vi "SiemensDigitalEnergyMeter.vi"() -> ()   [LabVIEW 2018, in "Visualization.lvlib" / "VisualizeSensor.lvclass"]
doc: "This VI listens for any measurement data associated with the provided PluginName and displays it to the user for analysis. The display is only suitable for data coming from the Siemens Plugin."
uses:
  VisualizeSensor.lvclass
  VisualizeBase/VisualizeBase_class/SubVIs/VisualizationOptions.ctl
  <vilib>/Utility/miscctls.llb/LVRectTypeDef.ctl
  Sensor/SensorShared/clSensorData.ctl
  <extravilib>/ChannelInstances/Tag-bool/Write With Abort.vi
  <extravilib>/ChannelInstances/Tag-bool/Read With Abort.vi
  <extravilib>/ChannelInstances/Tag-bool/Instantiate.vi
  <extravilib>/ChannelInstances/Tag-bool/EndpointRead.vi
  <vilib>/Utility/error.llb/Error Cluster From Error Code.vi
  <extravilib>/ChannelInstances/Tag-bool/Endpoint.vi
  <vilib>/ErrorRing/Error Ring.xnode
  <userlib>/NIST/NISTErrorLib/NISTErrorLib.lvlib
  VisualizeBase/VisualizeBase_class/VisualizeBase.lvclass
  Sensor/SensorShared/SensorShared.lvlib
  Sensor/SensorModule/SensorModule.lvlib
  <extravilib>/ChannelInstances/Tag-bool.lvlib
  TestClass/Test.lvclass
  StatusAndLog/VisualizeStatus.lvclass
panel:
  in  "btnPause":bool=TRUE
  out "VisualizationProperties":T1={"PauseAtStartup"=TRUE, "LogData"=FALSE, "LaunchInSubPanel"=TRUE, "FPMonitor"=0, "FPWindowBounds"={"Left"=0, "Top"=0, "Right"=0, "Bottom"=0}, "MonitorBounds"={"Left"=0, "Top"=0, "Right"=0, "Bottom"=0}}
  in  "INIFilePath":path
  in  "ModuleID":i32
  in  "Log Data":bool=TRUE
  in  "btnStop":bool
  in  "btnReset":bool
  in  "btnClearTest":bool
  out "Siemens":waveform(dbl)[](graph)=[{"t0"=timestamp(3657200531.6397257 s since 1904-01-01), "dt"=1.0, "Y"=[46.19]}, {"t0"=timestamp(3657200531.6397257 s since 1904-01-01), "dt"=1.0, "Y"=[2.0]}, {"t0"=timestamp(3657200531.6397257 s since 1904-01-01), "dt"=1.0, "Y"=[60.0]}]
  out "ErrorArray":errorcluster[](array[cluster])
  out "Incorrect DataType?":bool
  out "String Results":string="Sensor.RoomAlert1"
  in  "PluginName":string="Sensor.RoomAlert1"
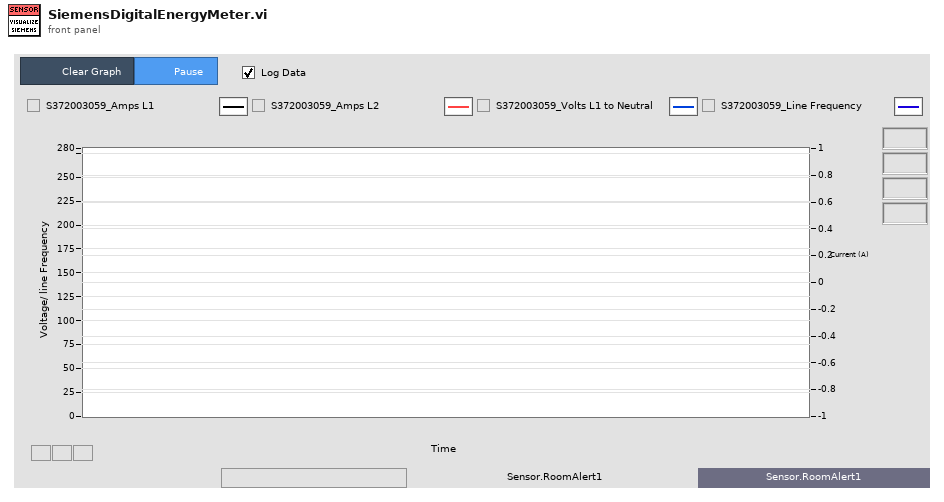
[diagram p1: front panel]
types:
  T1 = typedef "Visualization.lvlib/VisualizeBase.lvclass/VisualizationOptions.ctl" = cluster{"PauseAtStartup":bool, "LogData":bool, "LaunchInSubPanel":bool, "FPMonitor":u16, "FPWindowBounds":T2, "MonitorBounds":cluster{"Left":i16, "Top":i16, "Right":i16, "Bottom":i16}}
  T2 = typedef "LVRectTypeDef.ctl" = cluster{"Left":i16, "Top":i16, "Right":i16, "Bottom":i16}
  T3 = enum16{"open", "open or create", "create or replace", "create", "open (read-only)"}
  T4 = typedef "Visualization.lvlib/VisualizeBase.lvclass/VisRequestEvents.ctl" = cluster{"StopRequest":refnum<user-event>, "ResetRequest":refnum<user-event>, "FP Pop In or Out":refnum<user-event>}
  T5 = typedef "SensorShared.lvlib/clBroadcastEvents.ctl" = cluster{"DidInit":refnum<user-event>, "StatusUpdate":refnum<user-event>, "ErrorReport":refnum<user-event>, "DidStop":refnum<user-event>, "PathToINI":refnum<user-event>, "SensorReport":refnum<user-event>, "SensorConfig":refnum<user-event>}
  T6 = typedef "SensorShared.lvlib/clSensorData.ctl" = cluster{"SensorType":string, "SensorData":variant}
  T7 = typedef "Tag-bool.lvlib/))Channel.ctl" = refnum<queue>
  T8 = typedef "sizeaction.ctl" = enum32{"Minimized", "Maximized", "Resized"}
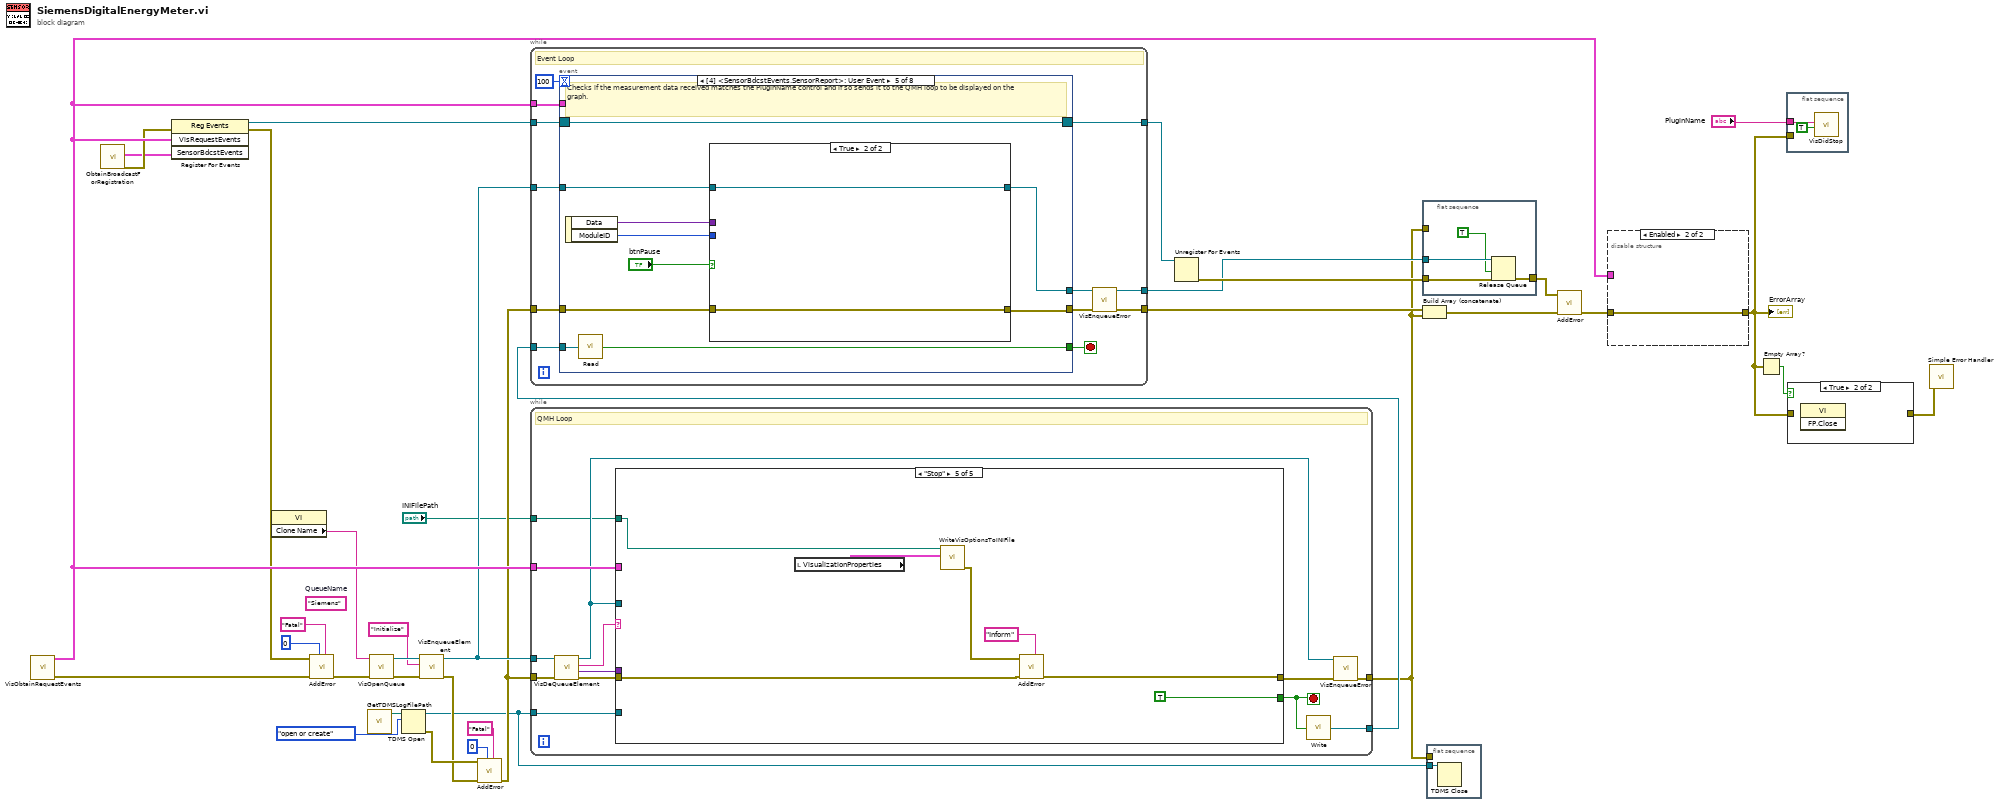
[diagram p0: block diagram]
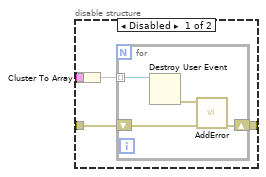
[diagram p2: hidden frame]
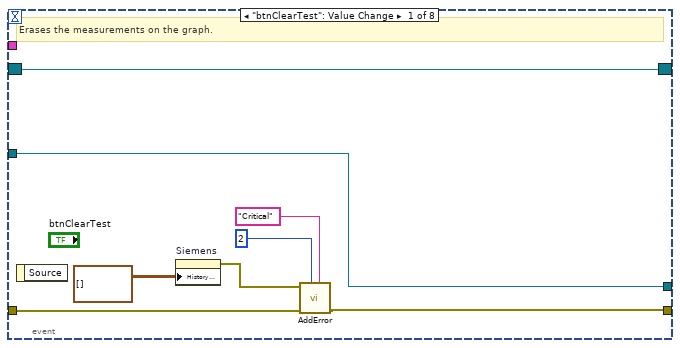
[diagram p3: hidden frame]
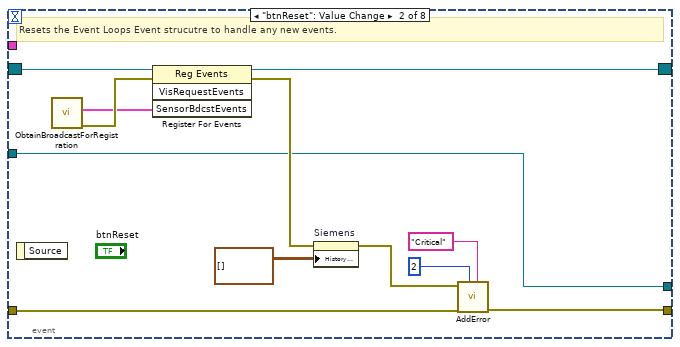
[diagram p4: hidden frame]
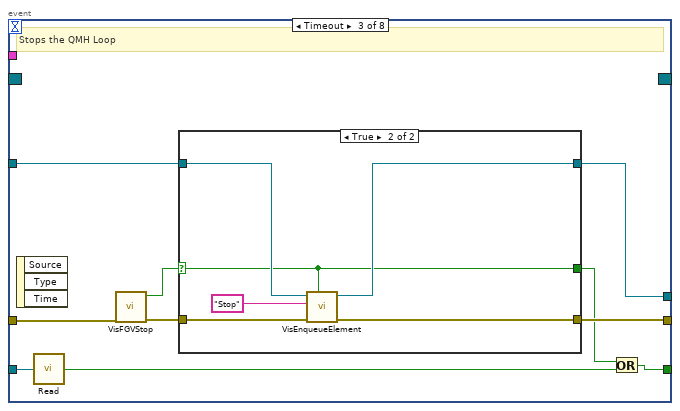
[diagram p5: hidden frame]
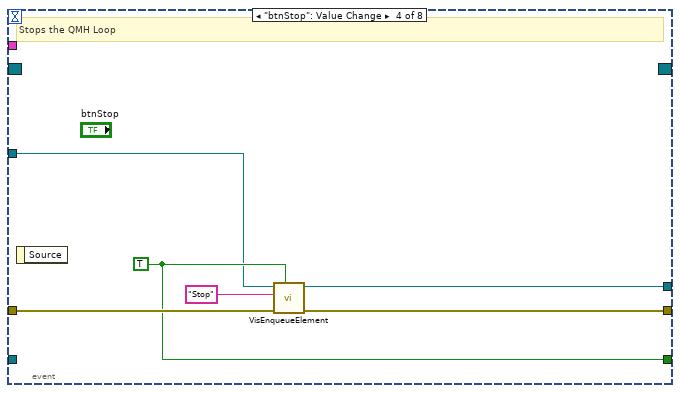
[diagram p7: hidden frame]
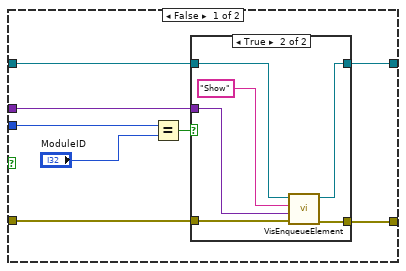
[diagram p8: hidden frame]
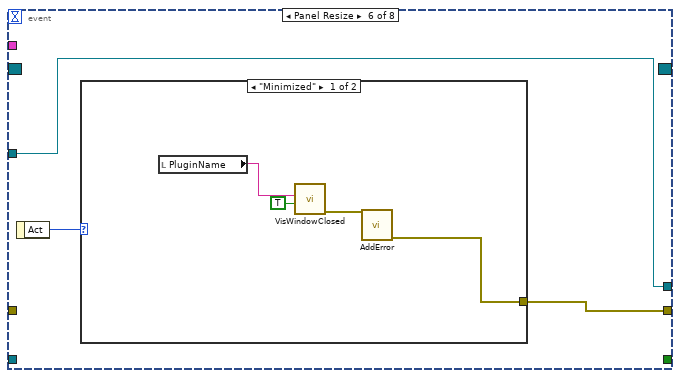
[diagram p10: hidden frame]
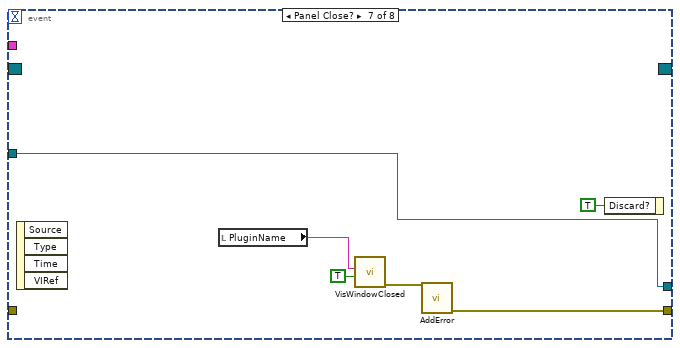
[diagram p12: hidden frame]
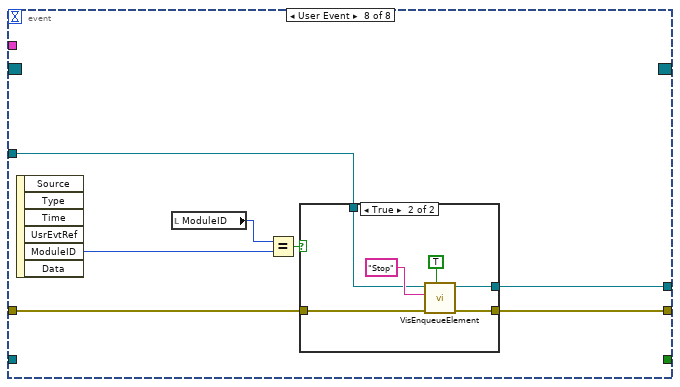
[diagram p13: hidden frame]
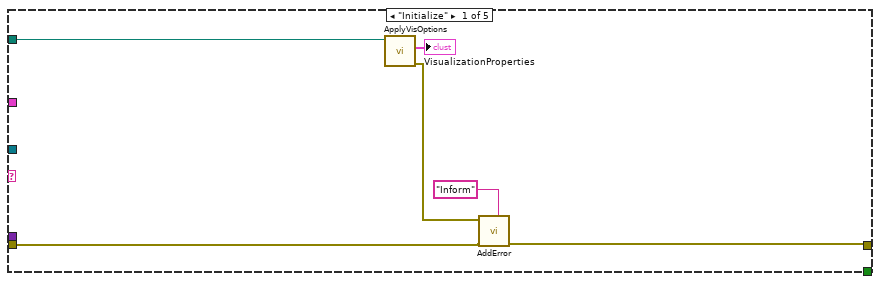
[diagram p15: hidden frame]
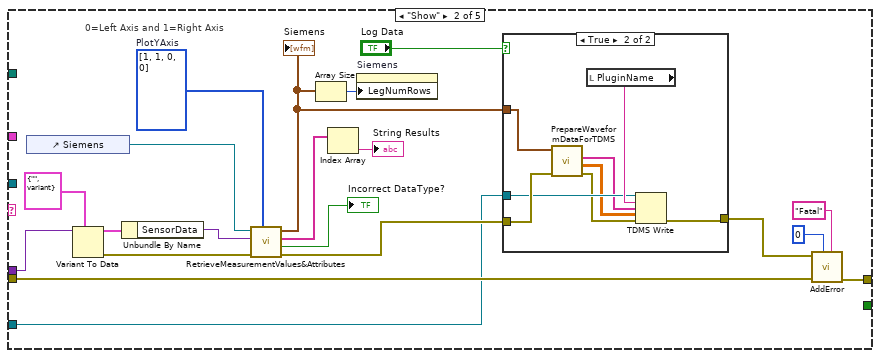
[diagram p16: hidden frame]
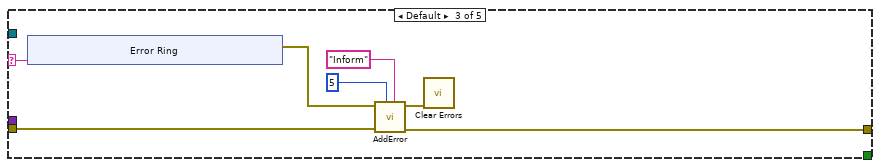
[diagram p18: hidden frame]
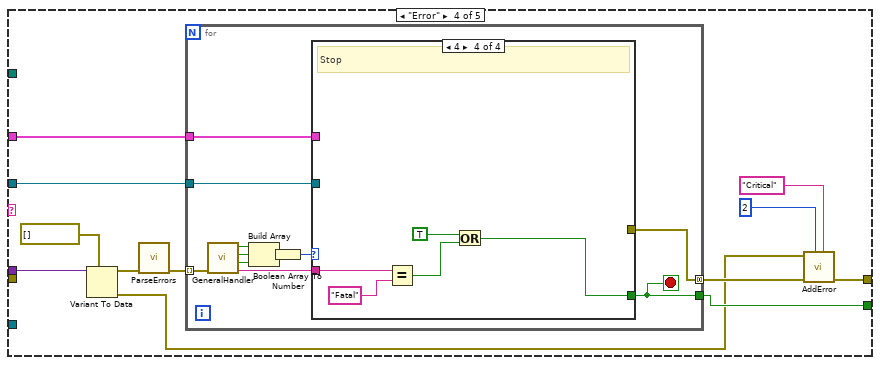
[diagram p19: hidden frame]
diagram:
  (unwired) "Siemens"  # QueueName
  n1 = call "VisObtainRequestEvents.vi"() -> ("Error"=w27:errorcluster[], "VisRequestEvents"=w29:T4)  [unwired: 10 in]
  n2 = call "ObtainBroadcastForRegistration.vi"() -> ("error out"=w23:errorcluster, "SensorBdcstEvents"=w15:T5)  [unwired: 10 in]
  n3 = register-events(error in=w23, w29, w15) -> (reference out=w36:refnum<event-registration>, error out=w26:errorcluster)  [unwired: 1 in]
  n4 = property class="VI"() -> ("Clone Name"=w13:string)  [unwired: 2 in, 2 out]
  n5 = call <userlib>:"AddError.vi"("Severity"="Fatal", "Priority"=u8 0, "ErrorArray In"=w27, "error in (no error)"=w26) -> ("ErrorArray Out"=w22:errorcluster[])  [unwired: 6 in, 1 out]
  n6 = call "GetTDMSLogFilePath.vi"() -> ("TDMS Log File Path"=w12:path)  [unwired: 11 in]
  n7 = call "VisOpenQueue.vi"("Error Array In"=w22, "QueueName"=w13) -> ("Error Array Out"=w20:errorcluster[], "queue out"=w21:refnum<queue>)  [unwired: 8 in]
  n8 = TDMS Open(10:T3."open or create" ("operation (0:open)"), 11:w12) -> (0:w8:errorcluster, 3:w5:refnum<k34>)  [unwired: 5 in]
  n9 = call "VisEnqueueElement.vi"("Error Array In"=w20, "Message"="Initialize", "queue in"=w21) -> ("Error Array Out"=w6:errorcluster[], "queue out"=w18:refnum<queue>)  [unwired: 7 in]
  n10 = call <userlib>:"AddError.vi"("Severity"="Fatal", "Priority"=u8 0, "ErrorArray In"=w6, "error in (no error)"=w8) -> ("ErrorArray Out"=w7:errorcluster[])  [unwired: 6 in, 1 out]
  n11 = while {
    tunnel: w7 -> [w43]
    tunnel: [w46] -> w4
    tunnel: w18 -> [w42]
    tunnel: w29 -> [w48]
    tunnel: [w39] -> w14
    tunnel: w5 -> [w38]
    tunnel: "INIFilePath" -> [w37]
    stop <- w49 stop-if-true
    # "QMH Loop"
    n12 = call "VisDeQueueElement.vi"("Error Array In"=w43, "Queue In"=w42) -> ("Error Array Out"=w41:errorcluster[], "Data"=w44:variant, "Message"=w45:string, "Queue Out"=w40:refnum<queue>)  [unwired: 6 in]
    n13 = case shown="\"Stop\"" w45 {
      selector: w45 -> [_ _ w91 _ _]
      tunnel: w44 -> [_ w69 _ w110 _]
      tunnel: w41 -> [w53 w73 w89 _ w135]
      tunnel: [w52 w75 w88 w100 w134] -> w47
      tunnel: [_ _ _ w106 TRUE] -> w49
      tunnel: w48 -> [_ _ _ w105 _]
      tunnel: w40 -> [_ _ _ w104 _]
      tunnel: w38 -> [_ w58 _ _ _]
      tunnel: w37 -> [w51 _ _ _ w133]
      frame "Initialize" {
        n14 = call "ApplyVisOptions.vi"("INIFilePath"=w51) -> ("error out"=w55:errorcluster, "VisualizationProperties"=→"VisualizationProperties":T1)  [unwired: 9 in]
        n15 = call <userlib>:"AddError.vi"("Severity"="Inform", "ErrorArray In"=w53, "error in (no error)"=w55) -> ("ErrorArray Out"=w52:errorcluster[])  [unwired: 7 in, 1 out]
      }
      frame "Show" {
        w66 = u32[] [1, 1, 0, 0]  # PlotYAxis
        # "0=Left Axis and 1=Right Axis"
        n16 = control-ref of="Siemens"() -> (w74:refnum<vi>)
        n17 = Variant To Data(type=T6 {"SensorType"="", "SensorData"=variant} ("clSensorData"), Variant=w69) -> (data=w67:T6, error out=w68:errorcluster)  [unwired: 1 in]
        n18 = Unbundle By Name(w67) -> ("SensorData"=w64:variant)
        n19 = call "RetrieveMeasurementValues&Attributes.vi"("PlotYScale"=w66, "error in (no error)"=w68, "Variant"=w64, "WaveformChartReference"=w74) -> ("error out"=w63:errorcluster, "Incorrect DataType?"=→"Incorrect DataType?":bool, "Array Of Strings"=w60:string[], "WaveformArrayOut"=w56:waveform(dbl)[])  [unwired: 3 in, 1 out]
        "Siemens" <- w56
        n20 = Array Size(array=w56) -> (size(s)=w57:i32)
        n21 = Index Array(array=w60) -> (element=→"String Results":string)  [unwired: 1 in]
        n22 = property on="Siemens" class="WFChart (strict)"("LegNumRows"=w57) -> ()  [unwired: 2 in, 2 out]
        n23 = case shown="True" "Log Data" {
          tunnel: w63 -> [w76 w84]
          tunnel: [w76 w82] -> w62
          tunnel: w56 -> [_ w79]
          tunnel: w58 -> [_ w81]
          frame False {
          }
          frame True {
            n24 = call "PrepareWaveformDataForTDMS.vi"("error in (no error)"=w84, "WaveformArray in"=w79) -> ("error out"=w80:errorcluster, "Measurement Data"=w77:dbl[][], "Channel Names"=w78:string[])  [unwired: 7 in]
            n25 = local read "PluginName"() -> (w83:string)
            n26 = TDMS Write(0:w81, 5:w83, 7:w78, 9:w77, 11:w80) -> (15:w82:errorcluster)  [unwired: 1 in, 3 out]
          }
        }
        n27 = call <userlib>:"AddError.vi"("Severity"="Fatal" ("String"), "Priority"=u8 0, "ErrorArray In"=w73, "error in (no error)"=w62) -> ("ErrorArray Out"=w75:errorcluster[])  [unwired: 6 in, 1 out]
      }
      frame Default {
        n28 = xnode "Error Ring"("parameter 0"=w91) -> ("error out"=w90:errorcluster)
        n29 = call <userlib>:"AddError.vi"("Severity"="Inform" ("String"), "Priority"=u8 5, "ErrorArray In"=w89, "error in (no error)"=w90) -> ("ErrorArray Out"=w88:errorcluster[], "error out"=w87:errorcluster)  [unwired: 6 in]
        n30 = call <vilib>:"Clear Errors.vi"("error in (no error)"=w87) -> ()  [unwired: 5 in, 2 out]
      }
      frame "Error" {
        n31 = Variant To Data(type=errorcluster[] [], Variant=w110) -> (data=w108:errorcluster[], error out=w99:errorcluster)  [unwired: 1 in]
        n32 = call <userlib>:"ParseErrors.vi"("ErrorArray"=w108) -> ("ErrorArray"=w107:errorcluster[])  [unwired: 8 in, 2 out]
        n33 = for {
          tunnel: w107 -> [w121] mode=indexing
          tunnel: [w115] -> w101 mode=concatenating
          tunnel: [w113] -> w106
          tunnel: w105 -> [w112]
          tunnel: w104 -> [w111]
          stop <- w113 stop-if-true
          n34 = call <userlib>:"GeneralHandler.vi"("error in (no error)"=w121) -> ("Severity"=w114:string, "Stop"=w118:bool, "Abort"=w119:bool, "Continue"=w120:bool)  [unwired: 6 in, 1 out]
          n35 = Build Array(w120, w119, w118) -> (w117:bool[])
          n36 = Boolean Array To Number(Boolean array=w117) -> (number=w116:u32)
          n37 = case shown="4" w116 {
            tunnel: [_ _ w126 _] -> w115
            tunnel: w114 -> [_ _ _ w131]
            tunnel: [_ _ _ w127] -> w113
            tunnel: w112 -> [_ _ _ _]
            tunnel: w111 -> [_ _ w122 _]
            frame 0, Default {
              # "No Dialog"
            }
            frame 1 {
              # "Continue"
            }
            frame 2 {
              # "Abort, Flush Queue"
              n38 = Flush Queue(queue=w122) -> (error out=w125:errorcluster)  [unwired: 1 in, 2 out]
              n39 = call <userlib>:"AddError.vi"("Severity"="Critical" ("String"), "Priority"=u8 1, "error in (no error)"=w125) -> ("ErrorArray Out"=w126:errorcluster[])  [unwired: 7 in, 1 out]
            }
            frame 4 {
              # "Stop"
              n40 = Equal?(x=w131, y="Fatal" ("x")) -> (x = y?=w128:bool)
              n41 = Or(x=TRUE, y=w128) -> (x .or. y?=w127:bool)
            }
          }
        }
        n42 = call <userlib>:"AddError.vi"("Severity"="Critical", "Priority"=u8 2, "ErrorArray In"=w101, "error in (no error)"=w99) -> ("ErrorArray Out"=w100:errorcluster[])  [unwired: 6 in, 1 out]
      }
      frame "Stop" {
        n43 = local read "VisualizationProperties"() -> (w132:T1)
        n44 = call "WriteVisOptionsToINIFile.vi"("Visualization Options"=w132, "INIFilePath"=w133) -> ("error out"=w136:errorcluster)  [unwired: 8 in, 1 out]
        n45 = call <userlib>:"AddError.vi"("Severity"="Inform", "ErrorArray In"=w135, "error in (no error)"=w136) -> ("ErrorArray Out"=w134:errorcluster[])  [unwired: 7 in, 1 out]
      }
    }
    n46 = call <extravilib>:"Write.vi"("element"=w49) -> ("channel"=w39:T7)  [unwired: 1 out]
    n47 = call "VisEnqueueError.vi"("Error Array In"=w47, "Queue in"=w40) -> ("Error Array Out"=w46:errorcluster[])  [unwired: 8 in, 1 out]
  }
  n48 = while {
    tunnel: w36 -> [w150]
    tunnel: [w144] -> w34
    tunnel: [w148] -> w35
    tunnel: w29 -> [w147]
    tunnel: w7 -> [w146]
    tunnel: w18 -> [w145]
    tunnel: [w141] -> w17
    tunnel: w14 -> [w139]
    stop <- w149 stop-if-true
    # "Event Loop"
    n49 = event shown="[4] <SensorBdcstEvents.SensorReport>: User Event" {
      selector: w150 -> [w152 w170 _ _ w201 _ _ _]
      dyn-events: [w152 w169 _ _ w201 _ _ _] -> w148
      timeout: 100 -> [_ _ _ _ _ _ _ _]
      tunnel: [_ _ w174 w192 w198 _ _ _] -> w149
      tunnel: [w155 w167 w176 w194 w203 w225 w232 w241] -> w143
      tunnel: w147 -> [_ _ _ _ _ _ _ _]
      tunnel: w146 -> [w156 w168 w177 w195 w204 _ _ w237]
      tunnel: w145 -> [w151 w160 w173 w190 w205 w224 w231 w240]
      tunnel: [w151 w160 w172 w193 w202 w224 w231 w242] -> w142
      tunnel: w139 -> [_ _ w180 _ w199 _ _ _]
      event "btnClearTest": Value Change {
        # "Erases the measurements on the graph."
        n50 = event-data() -> ()  [unwired: 1 in, 1 out]
        n51 = property on="Siemens" class="WFChart (strict)"("History Data"=waveform(dbl)[][] []) -> (error out=w154:errorcluster)  [unwired: 2 in, 1 out]
        n52 = call <userlib>:"AddError.vi"("Severity"="Critical", "Priority"=u8 2, "ErrorArray In"=w156, "error in (no error)"=w154) -> ("ErrorArray Out"=w155:errorcluster[])  [unwired: 6 in, 1 out]
      }
      event "btnReset": Value Change {
        # "Resets the Event Loops Event strucutre to handle any new events."
        n53 = event-data() -> ()  [unwired: 1 in, 1 out]
        n54 = call "ObtainBroadcastForRegistration.vi"() -> ("error out"=w161:errorcluster, "SensorBdcstEvents"=w159:T5)  [unwired: 10 in]
        n55 = register-events(reference=w170, error in=w161, w159) -> (reference out=w169:refnum<event-registration>, error out=w163:errorcluster)  [unwired: 1 in]
        n56 = property on="Siemens" class="WFChart (strict)"(error in=w163, "History Data"=waveform(dbl)[][] []) -> (error out=w162:errorcluster)  [unwired: 1 in, 1 out]
        n57 = call <userlib>:"AddError.vi"("Severity"="Critical", "Priority"=u8 2, "ErrorArray In"=w168, "error in (no error)"=w162) -> ("ErrorArray Out"=w167:errorcluster[])  [unwired: 6 in, 1 out]
      }
      event Timeout {
        # "Stops the QMH Loop"
        n58 = event-data() -> ()  [unwired: 1 in, 3 out]
        n59 = call <extravilib>:"Read.vi"("channel"=w180) -> ("element"=w175:bool)  [unwired: 1 in, 1 out]
        n60 = call "VisFGVStop.vi"("Error In"=w177) -> ("Error Out"=w178:errorcluster[], "Value"=w179:bool)  [unwired: 9 in]
        n61 = case shown="True" w179 {
          selector: w179 -> [w181 w184]
          tunnel: [w183 w187] -> w176
          tunnel: w178 -> [w183 w188]
          tunnel: w173 -> [w182 w186]
          tunnel: [w182 w185] -> w172
          tunnel: [w181 w184] -> w171
          frame False {
          }
          frame True {
            n62 = call "VisEnqueueElement.vi"("Priority? (F)"=w184, "Error Array In"=w188, "Message"="Stop", "queue in"=w186) -> ("Error Array Out"=w187:errorcluster[], "queue out"=w185:refnum<queue>)  [unwired: 6 in]
          }
        }
        n63 = Or(x=w171, y=w175) -> (x .or. y?=w174:bool)
      }
      event "btnStop": Value Change {
        w192 = TRUE ("Priority? (F)")
        # "Stops the QMH Loop"
        n64 = event-data() -> ()  [unwired: 1 in, 1 out]
        n65 = call "VisEnqueueElement.vi"("Priority? (F)"=w192, "Error Array In"=w195, "Message"="Stop", "queue in"=w190) -> ("Error Array Out"=w194:errorcluster[], "queue out"=w193:refnum<queue>)  [unwired: 6 in]
      }
      event User Event {
        # "Checks if the measurement data received matches the PluginName control and if so sends it to the QMH loop to be displayed on the graph."
        n66 = event-data() -> ("Data"=w200:variant, "ModuleID"=w197:i32)  [unwired: 1 in]
        n67 = call <extravilib>:"Read.vi"("channel"=w199) -> ("element"=w198:bool)  [unwired: 1 in, 1 out]
        n68 = case shown="True" "btnPause" {
          tunnel: w205 -> [w213 w223]
          tunnel: w204 -> [w212 w222]
          tunnel: [w211 w222] -> w203
          tunnel: [w210 w223] -> w202
          tunnel: w200 -> [w209 _]
          tunnel: w197 -> [w206 _]
          frame False {
            n69 = Equal?(x=w206, y="ModuleID") -> (x = y?=w208:bool)
            n70 = case shown="True" w208 {
              tunnel: [w214 w220] -> w211
              tunnel: w213 -> [w215 w219]
              tunnel: w212 -> [w214 w221]
              tunnel: [w215 w217] -> w210
              tunnel: w209 -> [_ w218]
              frame False {
              }
              frame True {
                n71 = call "VisEnqueueElement.vi"("Error Array In"=w221, "Data"=w218, "Message"="Show", "queue in"=w219) -> ("Error Array Out"=w220:errorcluster[], "queue out"=w217:refnum<queue>)  [unwired: 6 in]
              }
            }
          }
          frame True {
          }
        }
      }
      event Panel Resize {
        n72 = event-data() -> ("Act"=w226:T8)  [unwired: 1 in]
        n73 = case shown="\"Minimized\"" w226 {
          tunnel: [w227 _] -> w225
          frame "Minimized" {
            n74 = local read "PluginName"() -> (w229:string)
            n75 = call "VisWindowClosed.vi"("Window Closed?"=TRUE ("Window Minimized or Clozed?"), "Module Name"=w229) -> ("error out"=w230:errorcluster)  [unwired: 9 in]
            n76 = call <userlib>:"AddError.vi"("error in (no error)"=w230) -> ("ErrorArray Out"=w227:errorcluster[])  [unwired: 9 in, 1 out]
          }
          frame "Maximized", Default {
          }
        }
      }
      event Panel Close? {
        n77 = event-data() -> ()  [unwired: 1 in, 4 out]
        n78 = local read "PluginName"() -> (w233:string)
        n79 = call "VisWindowClosed.vi"("Window Closed?"=TRUE ("Window Minimized or Clozed?"), "Module Name"=w233) -> ("error out"=w235:errorcluster)  [unwired: 9 in]
        n80 = call <userlib>:"AddError.vi"("error in (no error)"=w235) -> ("ErrorArray Out"=w232:errorcluster[])  [unwired: 9 in, 1 out]
        n81 = event-data("Discard?"=TRUE) -> ()  [unwired: 1 in, 1 out]
      }
      event User Event {
        n82 = event-data() -> ("ModuleID"=w239:i32)  [unwired: 1 in, 5 out]
        n83 = local read "ModuleID"() -> (w238:i32)
        n84 = Equal?(x=w238, y=w239) -> (x = y?=w243:bool)
        n85 = case shown="True" w243 {
          tunnel: [w244 w249] -> w241
          tunnel: [w245 w248] -> w242
          tunnel: w240 -> [w245 w247]
          tunnel: w237 -> [w244 w246]
          frame False {
          }
          frame True {
            n86 = call "VisEnqueueElement.vi"("Priority? (F)"=TRUE, "Error Array In"=w246, "Message"="Stop", "queue in"=w247) -> ("Error Array Out"=w249:errorcluster[], "queue out"=w248:refnum<queue>)  [unwired: 6 in]
          }
        }
      }
    }
    n87 = call "VisEnqueueError.vi"("Error Array In"=w143, "Queue in"=w142) -> ("Error Array Out"=w144:errorcluster[], "Queue out"=w141:refnum<queue>)  [unwired: 8 in]
  }
  n88 = Unregister For Events(event registration refnum=w35) -> (error out=w33:errorcluster)  [unwired: 1 in]
  n89 = flat-sequence {
    tunnel: w33 -> [w255]
    tunnel: [w254] -> w31
    tunnel: w17 -> [w253]
    tunnel: w4 -> [_]
    frame #0 {
      n90 = Release Queue(queue=w253, force destroy? (F)=TRUE, error in (no error)=w255) -> (error out=w254:errorcluster)  [unwired: 2 out]
    }
  }
  n91 = Build Array (concatenate)(w34, w4) -> (w32:errorcluster[])
  n92 = flat-sequence {
    tunnel: w5 -> [w256]
    tunnel: w4 -> [_]
    frame #0 {
      n93 = TDMS Close(11:w256) -> ()  [unwired: 1 in, 2 out]
    }
  }
  n94 = call <userlib>:"AddError.vi"("ErrorArray In"=w32, "error in (no error)"=w31) -> ("ErrorArray Out"=w30:errorcluster[])  [unwired: 8 in, 1 out]
  n95 = disable-structure shown="Enabled" {
    disable-tunnel: w30 -> [w259 w265]
    disable-tunnel: w29 -> [w258 _]
    disable-tunnel: [w257 w265] -> w1
    frame Disabled {
      n96 = Cluster To Array(cluster=w258) -> (array=w260:refnum<user-event>[])
      n97 = for {
        tunnel: w260 -> [w264] mode=indexing
        shift-right: [w263] -> w257
        shift-left: w259 -> [w262]
        n98 = Destroy User Event(user event=w264) -> (error out=w261:errorcluster)  [unwired: 1 in]
        n99 = call <userlib>:"AddError.vi"("ErrorArray In"=w262, "error in (no error)"=w261) -> ("ErrorArray Out"=w263:errorcluster[])  [unwired: 8 in, 1 out]
      }
    }
    frame Enabled {
    }
  }
  "ErrorArray" <- w1
  n100 = Empty Array?(array=w1) -> (empty?=w28:bool)
  n101 = flat-sequence {
    tunnel: "PluginName" -> [w267]
    tunnel: w1 -> [_]
    frame #0 {
      n102 = call "VisDidStop.vi"("DidStop?"=TRUE, "Module Name"=w267) -> ()  [unwired: 9 in, 1 out]
    }
  }
  n103 = case shown="True" w28 {
    tunnel: [w268 _] -> w16
    tunnel: w1 -> [w269 _]
    frame False {
      n104 = Merge Errors(w269) -> (w268:errorcluster)
    }
    frame True {
      n105 = invoke class="VI" method="FP.Close"() -> ()  [unwired: 3 in, 3 out]
    }
  }
  n106 = call <vilib>:"Simple Error Handler.vi"("error in (no error)"=w16) -> ()  [unwired: 4 in, 5 out]
